vi "remove_string_duplicates.vi"(11 "In":string[](array[string])=["A", "A", "A"]) -> (3 "Out":string[](array[string]))   [LabVIEW 2017]
doc: "Use this VI to remove duplicate, adjacent elements from an array. To use this VI, enter values in the \"In\" array and run."
panel:
  # "Select Help»Show Context Help and move the cursor over the VI icon to display help for this VI."
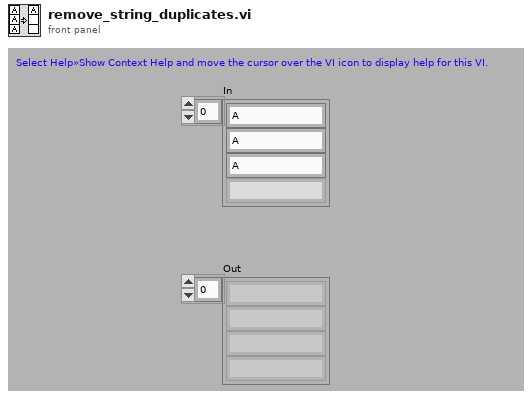
[diagram p1: front panel]
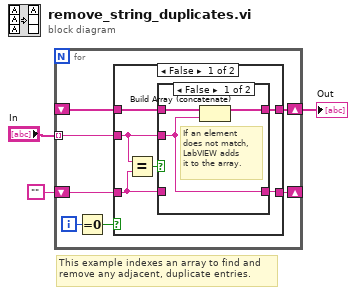
[diagram p0: block diagram]
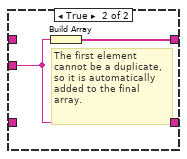
[diagram p3: hidden frame]
diagram:
  # "This example indexes an array to find and\nremove any adjacent, duplicate entries."
  n1 = for {
    tunnel: "In" -> [w8] mode=indexing
    shift-right: [w6] -> _
    shift-left: "" -> [w5]
    shift-right: [w7] -> w2
    shift-left: _ -> [w4]
    i -> [w10]
    n2 = Equal To 0?(x=w10) -> (x = 0?=w9:bool)
    n3 = case shown="False" w9 {
      tunnel: w8 -> [w13 w22]
      tunnel: [w14 w23] -> w7
      tunnel: [w16 w22] -> w6
      tunnel: w5 -> [w12 _]
      tunnel: w4 -> [w15 _]
      frame False {
        n4 = Equal?(x=w13, y=w12) -> (x = y?=w11:bool)
        n5 = case shown="False" w11 {
          tunnel: w12 -> [_ w21]
          tunnel: [w17 w21] -> w16
          tunnel: [w18 w20] -> w14
          tunnel: w15 -> [w19 w20]
          tunnel: w13 -> [w17 _]
          frame False {
            # "If an element\ndoes not match,\nLabVIEW adds\nit to the array."
            n6 = Build Array (concatenate)(w19, w17) -> (w18:string[])
          }
          frame True {
            # "If an element\nmatches the\none before it,\nit is not added\nto the array."
          }
        }
      }
      frame True {
        # "The first element\ncannot be a duplicate,\nso it is automatically\nadded to the final\narray."
        n7 = Build Array(w22) -> (w23:string[])
      }
    }
  }
  "Out" <- w2
